vi "Create_Plot.vi"(1 "First Graph":T2) -> (0 "Array":cluster{"X array":dbl[], "Y array":dbl[]}[](array[cluster]))   [LabVIEW 2016]
uses:
  Controls/Graph_Type.ctl
  Globals/Meas_global.vi
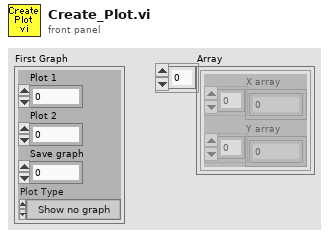
[diagram p1: front panel]
types:
  T1 = typedef "Graph_Type.ctl" = enum16{"Show no graph", "Voltage trace", "Velocity trace", "Vel histogram", "Spectrum", "f.E(f) v Log f", "Auto-Corr"}
  T2 = cluster{"Plot 1":u16, "Plot 2":u16, "Save graph":u16, "Plot Type":T1}
  T3 = enum16{"Save no data", "Save data in new files", "Save data in existing files"}
  T4 = typedef "Time_Trace_Cluster.ctl" = cluster{"Weighting":dbl[], "Time (s)":dbl[], "Voltage":dbl[], "Eng Values":dbl[]}
  T5 = typedef "XY_Plot_Cluster.ctl" = cluster{"First Name":string, "Second Name":string, "X axis name":string, "Y axis name":string, "X array":dbl[], "Y array":dbl[], "Weighting":dbl[]}
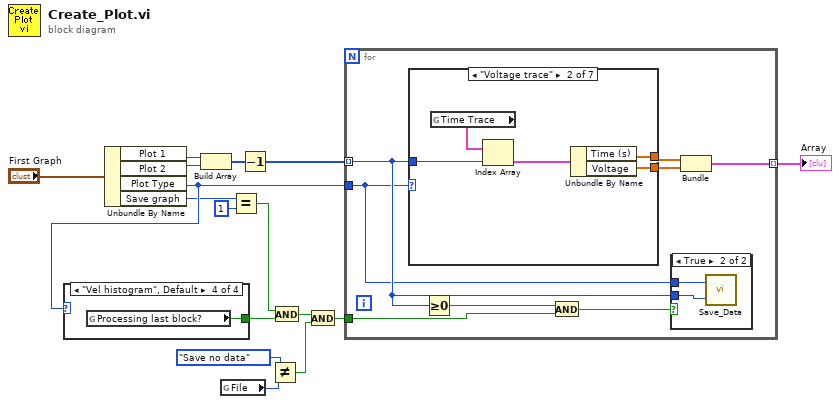
[diagram p0: block diagram]
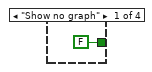
[diagram p2: hidden frame]
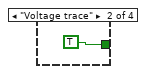
[diagram p3: hidden frame]
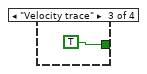
[diagram p4: hidden frame]
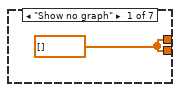
[diagram p6: hidden frame]
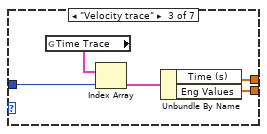
[diagram p7: hidden frame]
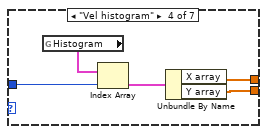
[diagram p8: hidden frame]
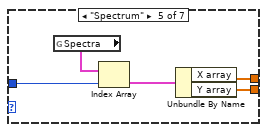
[diagram p9: hidden frame]
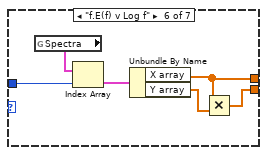
[diagram p10: hidden frame]
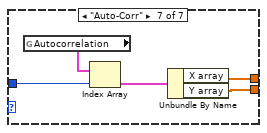
[diagram p11: hidden frame]
diagram:
  n1 = Unbundle By Name("First Graph") -> ("Plot 1"=w7:u16, "Plot 2"=w8:u16, "Plot Type"=w15:T1, "Save graph"=w12:u16)
  n2 = case shown="\"Vel histogram\", Default" w15 {
    tunnel: [FALSE TRUE TRUE w20] -> w16
    frame "Show no graph" {
    }
    frame "Voltage trace" {
    }
    frame "Velocity trace" {
    }
    frame "Vel histogram", Default {
      n3 = global read "Meas_global.vi" "Processing last block?"() -> (w20:bool)
    }
  }
  n4 = Build Array(w7, w8) -> (w9:u16[])
  n5 = global read "Meas_global.vi" "File"() -> (w2:T3)
  n6 = Equal?(x=w12, y=u16 1 ("Save graph")) -> (x = y?=w14:bool)
  n7 = Decrement(x=w9) -> (x-1=w6:u16[])
  n8 = Not Equal?(x=T3."Save no data" ("File"), y=w2) -> (x != y?=w1:bool)
  n9 = And(x=w14, y=w16) -> (x .and. y?=w5:bool)
  n10 = And(x=w5, y=w1) -> (x .and. y?=w4:bool)
  n11 = for {
    tunnel: w6 -> [w23] mode=indexing
    tunnel: w15 -> [w22]
    tunnel: [w28] -> w11 mode=indexing
    tunnel: w4 -> [w24]
    n12 = case shown="\"Voltage trace\"" w22 {
      tunnel: [w31 w32 w37 w46 w51 w57 w62] -> w27
      tunnel: [w31 w36 w41 w45 w50 w55 w61] -> w26
      tunnel: w23 -> [_ w33 w39 w44 w49 w54 w59]
      frame "Show no graph" {
        w31 = dbl[] [] ("X array")
      }
      frame "Voltage trace" {
        n13 = global read "Meas_global.vi" "Time Trace"() -> (w35:T4[])
        n14 = Index Array(array=w35, index=w33) -> (element=w34:T4)
        n15 = Unbundle By Name(w34) -> ("Time (s)"=w32:dbl[], "Voltage"=w36:dbl[])
      }
      frame "Velocity trace" {
        n16 = global read "Meas_global.vi" "Time Trace"() -> (w40:T4[])
        n17 = Index Array(array=w40, index=w39) -> (element=w38:T4)
        n18 = Unbundle By Name(w38) -> ("Time (s)"=w37:dbl[], "Eng Values"=w41:dbl[])
      }
      frame "Vel histogram" {
        n19 = global read "Meas_global.vi" "Histogram"() -> (w42:T5[])
        n20 = Index Array(array=w42, index=w44) -> (element=w43:T5)
        n21 = Unbundle By Name(w43) -> ("X array"=w46:dbl[], "Y array"=w45:dbl[])
      }
      frame "Spectrum" {
        n22 = global read "Meas_global.vi" "Spectra"() -> (w47:T5[])
        n23 = Index Array(array=w47, index=w49) -> (element=w48:T5)
        n24 = Unbundle By Name(w48) -> ("X array"=w51:dbl[], "Y array"=w50:dbl[])
      }
      frame "f.E(f) v Log f" {
        n25 = global read "Meas_global.vi" "Spectra"() -> (w53:T5[])
        n26 = Index Array(array=w53, index=w54) -> (element=w52:T5)
        n27 = Unbundle By Name(w52) -> ("X array"=w57:dbl[], "Y array"=w56:dbl[])
        n28 = Multiply(x=w57, y=w56) -> (x*y=w55:dbl[])
      }
      frame "Auto-Corr" {
        n29 = global read "Meas_global.vi" "Autocorrelation"() -> (w60:T5[])
        n30 = Index Array(array=w60, index=w59) -> (element=w58:T5)
        n31 = Unbundle By Name(w58) -> ("X array"=w62:dbl[], "Y array"=w61:dbl[])
      }
    }
    n32 = Greater Or Equal To 0?(x=w23) -> (x >= 0?=w25:bool)
    n33 = And(x=w25, y=w24) -> (x .and. y?=w21:bool)
    n34 = case shown="True" w21 {
      tunnel: w22 -> [_ w30]
      tunnel: w23 -> [_ w29]
      frame False {
      }
      frame True {
        n35 = call "Save_Data.vi"("Index"=w29, "Plot Type"=w30) -> ()  [unwired: 1 in]
      }
    }
    n36 = Bundle("X array"=w27, "Y array"=w26) -> (w28:cluster{"X array":dbl[], "Y array":dbl[]})  [unwired: 1 in]
  }
  "Array" <- w11
